vi "Read Session.vi"(8 "Error In":errorcluster, 11 "Listener In":refnum<class "Listener.lvclass">) -> (0 "Error Out":errorcluster, 2 "Session":refnum<class "Session.lvclass">, 3 "Listener Out":refnum<class "Listener.lvclass">)   [LabVIEW 2018, in "Toolkit.lvlib" / "Listener.lvclass"]
uses:
  Listener.lvclass
  Session/Session.lvclass
  Listener.lvclass/Listener.ctl
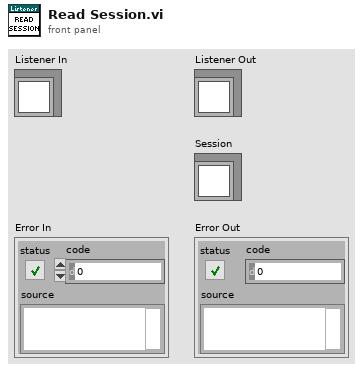
[diagram p1: front panel]
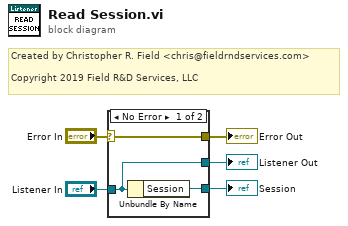
[diagram p0: block diagram]
diagram:
  # "Created by Christopher R. Field <chris@fieldrndservices.com>\n\nCopyright 2019 Field R&D Services, LLC"
  n1 = case shown="No Error" "Error In" {
    selector: "Error In" -> [w7 w10]
    tunnel: "Listener In" -> [w8 w9]
    tunnel: [w8 w9] -> w2
    tunnel: [w7 w10] -> w4
    tunnel: [w6 _] -> w1
    frame No Error {
      n2 = Unbundle By Name(w8) -> ("Session"=w6:refnum<class "Session.lvclass">)
    }
    frame Error {
    }
  }
  "Error Out" <- w4
  "Listener Out" <- w2
  "Session" <- w1
